vi "SaveDataFile.vi"(0 "Data Array":dbl[][](array[numeric]), 1 "Temperature":dbl, 3 "Humidity":dbl, 5 "no. of arrays":i32, 9 "Actual array lengths":i32, 11 "Error In":errorcluster, 12 "Array Titles":string, 13 "Strip Segment":string, 14 "Arrays format":string) -> (4 "Filename OUT":string, 6 "Pathname OUT":string, 10 "Path + Filename OUT":string, 15 "Error Out":errorcluster)   [LabVIEW 2013]
uses:
  globals/QC_RunInformation.vi
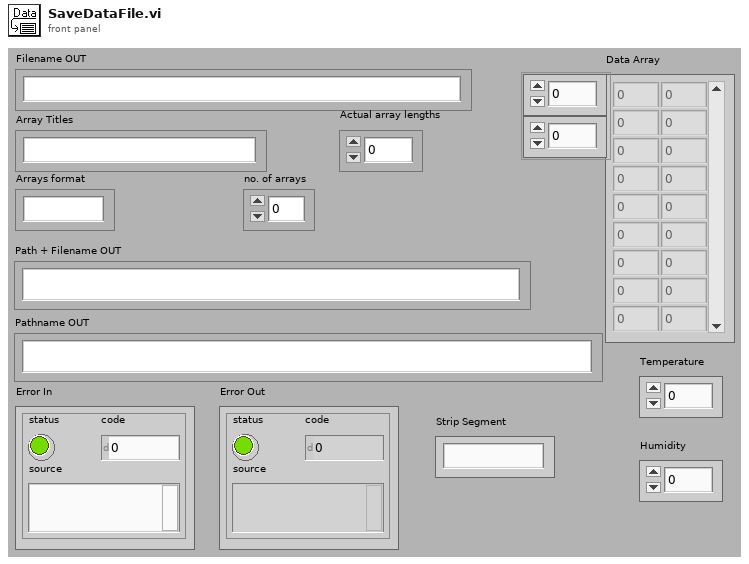
[diagram p1: front panel]
types:
  T1 = enum16{"open", "open or create", "create or replace", "create"}
  T2 = cluster{"Institute":string, "Manufacturers":string[], "Devices":string[], "Serialnumbers Lookup DB":string, "Data directory":string, "Backup & screenshot directory":string, "List of known users":string[], "Measurement switch not used":bool, "Measurement Switch":string, "DUT Switch":string}
  T3 = cluster{"Sensor Serial No.:":string, "Wafer Serial No.:":string, "Batch:":string, "Manufacturer:":string, "Device Category:":string, "Database Serial No.:":string, "Date Initiated:":string, "Time Initiated:":string, "Test":string, "Instruments used:":string, "Probeplan used:":string, "End of Run comment:":string, "User:":string}
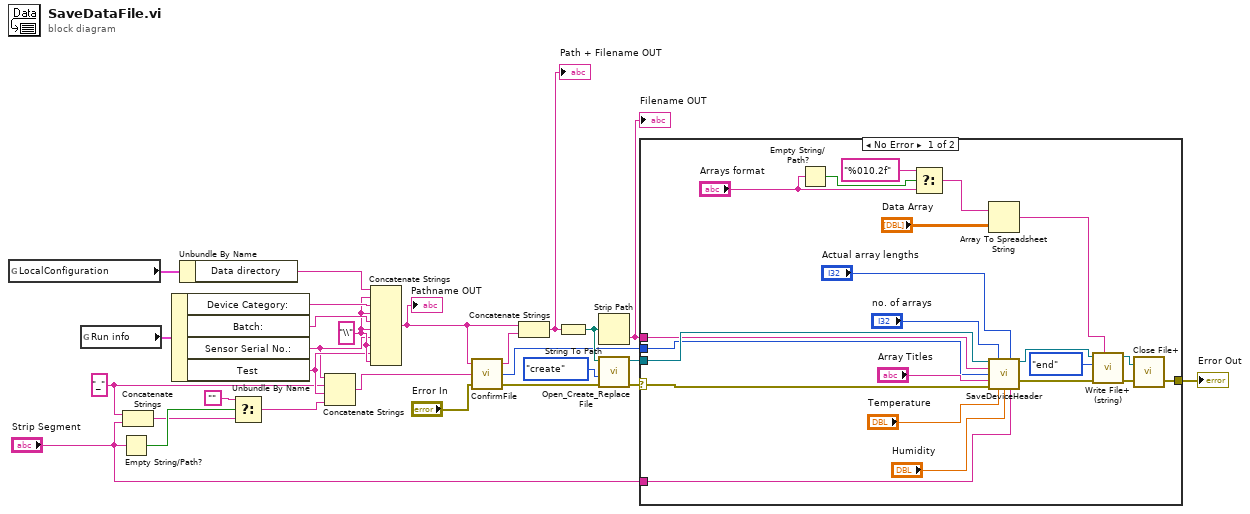
[diagram p0: block diagram]
diagram:
  w6 = "_"
  w17 = "\\"
  n1 = global read "QC_RunInformation.vi" "LocalConfiguration"() -> (w27:T2)
  n2 = global read "QC_RunInformation.vi" "Run info"() -> (w26:T3)
  n3 = Empty String/Path?(string/path="Strip Segment") -> (empty?=w8:bool)
  n4 = Concatenate Strings(w6, "Strip Segment") -> (w4:string)
  n5 = Unbundle By Name(w26) -> ("Device Category:"=w24:string, "Batch:"=w23:string, "Sensor Serial No.:"=w3:string, "Test"=w15:string)
  n6 = Unbundle By Name(w27) -> ("Data directory"=w25:string)
  n7 = Select(t="", s=w8, f=w4) -> (s? t:f=w5:string)
  n8 = Concatenate Strings(w3, w6, w15, w5) -> (w16:string)
  n9 = Concatenate Strings(w25, w17, w24, w17, w23, w17, w3, w17, w15, w17) -> (w11:string)
  "Pathname OUT" <- w11
  n10 = call "ConfirmFile.vi"("Error In"="Error In", "Filename IN"=w16, "Pathname IN"=w11) -> ("Error Out"=w12:errorcluster, "Run Number"=w2:i32, "Filename:"=w10:string)
  n11 = Concatenate Strings(w11, w10) -> (w9:string)
  "Path + Filename OUT" <- w9
  n12 = String To Path(string=w9) -> (path=w19:path)
  n13 = Strip Path(path=w19) -> (name=w20:string)  [unwired: 1 out]
  "Filename OUT" <- w20
  n14 = call <vilib>:"Open_Create_Replace File.vi"("error in (no error)"=w12, "function (open:0)"=T1."create", "file path"=w19) -> ("error out"=w18:errorcluster, "refnum"=w21:refnum<file>)  [unwired: 5 in, 2 out]
  n15 = case shown="No Error" w18 {
    selector: w18 -> [w49 w50]
    tunnel: w21 -> [w38 _]
    tunnel: w20 -> [w37 _]
    tunnel: [w33 w50] -> w14
    tunnel: w2 -> [w29 _]
    tunnel: "Strip Segment" -> [w28 _]
    frame No Error {
      n16 = Empty String/Path?(string/path="Arrays format") -> (empty?=w46:bool)
      n17 = Select(t="%010.2f", s=w46, f="Arrays format") -> (s? t:f=w44:string)
      n18 = Array To Spreadsheet String(array="Data Array", 3:w44) -> (spreadsheet string=w43:string)  [unwired: 1 in]
      n19 = call "SaveDeviceHeader.vi"("File Refnum in"=w38, "no. of arrays"="no. of arrays", "Array Lengths"="Actual array lengths", "Filename"=w37, "Run Number"=w29, "Array Titles"="Array Titles", "error in (no error)"=w49, "Temperature"="Temperature", "Humidity"="Humidity", "Strip Segment"=w28) -> ("File Refnum out"=w39:refnum<file>, "error out"=w30:errorcluster)  [unwired: 3 in, 1 out]
      n20 = call <vilib>:"Write File+ (string).vi"("string"=w43, "error in (no error)"=w30, "pos mode (rel. to end:1)"=enum16{"start", "end", "current"}."end", "refnum"=w39) -> ("error out"=w42:errorcluster, "dup refnum"=w40:refnum<file>)  [unwired: 3 in, 1 out]
      n21 = call <vilib>:"Close File+.vi"("error in (no error)"=w42, "refnum"=w40) -> ("error out"=w33:errorcluster)  [unwired: 3 in, 2 out]
    }
    frame Error {
    }
  }
  "Error Out" <- w14
